vi "User Event star.vi"(8 "error in":errorcluster, 9 "event data":bool, 11 "Function":enum16{"Open", "Event Write", "Close"}(ring)) -> (0 "error out":errorcluster, 3 "Star Event":refnum<user-event>)   [LabVIEW 2016]
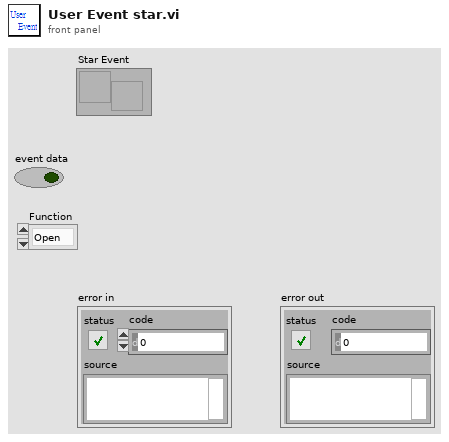
[diagram p1: front panel]
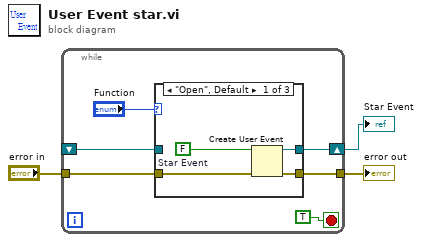
[diagram p0: block diagram]
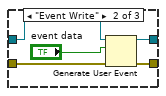
[diagram p2: hidden frame]
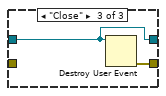
[diagram p3: hidden frame]
diagram:
  n1 = while {
    shift-right: [w7] -> w1
    shift-left: _ -> [w6]
    tunnel: "error in" -> [w5]
    tunnel: [w4] -> w2
    stop <- TRUE stop-if-true
    n2 = case shown="\"Open\", Default" "Function" {
      tunnel: [w12 w17 w19] -> w7
      tunnel: w6 -> [_ w18 w19]
      tunnel: w5 -> [w10 w15 _]
      tunnel: [w11 w14 w20] -> w4
      frame "Open", Default {
        w13 = FALSE  # Star Event
        n3 = Create User Event(user event datatype=w13, error in=w10) -> (user event=w12:refnum<user-event>, error out=w11:errorcluster)
      }
      frame "Event Write" {
        n4 = Generate User Event(user event=w18, event data cluster="event data", error in=w15) -> (user event out=w17:refnum<user-event>, error out=w14:errorcluster)  [unwired: 1 in]
      }
      frame "Close" {
        n5 = Destroy User Event(user event=w19) -> (error out=w20:errorcluster)  [unwired: 1 in]
      }
    }
  }
  "error out" <- w2
  "Star Event" <- w1
